vi "PH_SHS_Analysis.PC Set SHS Device Config.vi"(0 "i ref in":refnum<vi>, 2 "SHS Device Config":T1 {"wavelength [m]" format="%#_6p"; "pixel size [m/px]" format="%#_6p"; "focal length [m]" format="%#_6p"}, 5 "error IO":errorcluster) -> (14 "i ref out":refnum<vi>, 19 "error out":errorcluster)   [LabVIEW 2014, in "PH_SHS_Analysis.lvlib"]
uses:
  PH_SHS_Analysis.lvlib
  CSlibraries-extern/shs/SHS_Analysis/SHS_DeviceConfig.ctl
  CSlibraries-extern/shs/SHS_Analysis/SHS_Analysis.lvlib
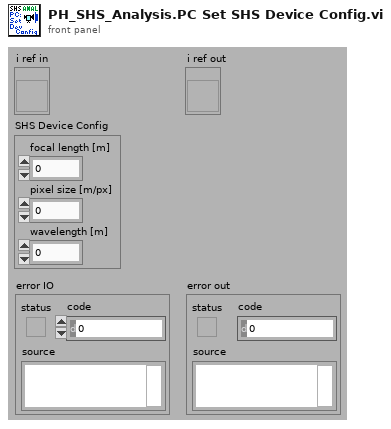
[diagram p1: front panel]
types:
  T1 = typedef "SHS_Analysis.lvlib/SHS_DeviceConfig.ctl" = cluster{"focal length [m]":dbl, "pixel size [m/px]":dbl, "wavelength [m]":dbl}
  T2 = typedef "PH_SHS_Analysis.lvlib/PH_SHS_Analysis.i attribute.ctl" = cluster{"GUI Refs":cluster{"Delete":refnum<vi>, "Global On":refnum<vi>, "Cam Source":refnum<vi>, "Calibration Data File":refnum<vi>, "Calibration status":refnum<vi>, "Show overlay":refnum<vi>, "SHS Device Config":refnum<vi>, "Result":refnum<vi>, "Consider Tilt":refnum<vi>, "Working Reference":refnum<vi>, "Remove Tilt":refnum<vi>, "Take Cali  Reference":refnum<vi>, "Publishing Data Status":refnum<vi>, "Calibration Data":refnum<vi>}, "Calibration":cluster{"Status":T3, "Data":T4, "File":path}, "Result":T9, "Image":T12, "SHS Device Config":T1, "Show Overlay":bool, "GradientZernikeMatrix":dbl[][], "Consider Tilt":bool, "Working Reference":T5, "Zernicke Service ID":i32, "PSDB Image":T12}
  T3 = typedef "PH_StatusHandler.lvlib/PH_StatusHandler.Status.ctl" = i16
  T4 = typedef "PH_SHS_Analysis_Calibrator.lvlib/PH_SHS_Analysis_Calibrator.Analysis Calibration Data.ctl" = cluster{"Date":string, "Time":string, "Cam Settings":cluster{"Cam ID":string, "Gain":dbl, "Brightness":dbl, "Shutter":dbl, "Cam Error":bool, "Mode":i32}, "SHS Reference Result":T5, "Pixel Size":dbl, "MLA Pitch":dbl, "Method":enum16{"automatic", "manual"}, "Calibration Data calculated":bool, "No Problems at calculation?":bool, "error out":errorcluster}
  T5 = typedef "SHS_Common.lvlib/SHSReference.ctl" = cluster{"Reference":T6[][], "Lens Array Pitch [px]":dbl}
  T6 = typedef "SHS_Common.lvlib/ReferencePoint.ctl" = cluster{"Rect":T7, "Point":T8}
  T7 = typedef "SHS_Common.lvlib/Rectangle.ctl" = cluster{"Left":i32, "Top":i32, "Right":i32, "Bottom":i32}
  T8 = typedef "SHS_Common.lvlib/Point.ctl" = cluster{"x":dbl, "y":dbl, "valid?":bool, "weight":dbl}
  T9 = typedef "PH_SHS_Analysis.lvlib/PH_SHS_Analysis.Result.ctl" = cluster{"Time Stamp":timestamp, "Zernike Coefficients":T10, "PtV [lambda]":dbl, "Shifts":T11, "Measurement Quality":cluster{dbl, dbl, dbl}, "Measurement valid?":bool}
  T10 = typedef "PH_SHS_Analysis.lvlib/PH_SHS_Analysis.Zernike Coefficients.ctl" = cluster{"Tilt x":dbl, "Tilt y":dbl, "Defocus":dbl, "Astig 0°":dbl, "Astig 45°":dbl, "Coma x":dbl, "Coma y":dbl, "Spherical":dbl, "Trefoil 0°":dbl, "Trefoil 30°":dbl, "2nd Astig 0°":dbl, "2nd Astig 45°":dbl, "2nd Coma x":dbl, "2nd Coma y":dbl, "2nd Spherical":dbl}
  T11 = typedef "SHS_Common.lvlib/Shifts.ctl" = T8[][]
  T12 = typedef "IMAQ Image.ctl" = refnum<image>
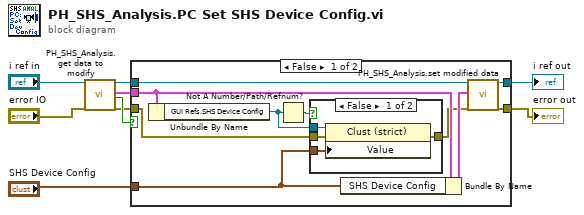
[diagram p0: block diagram]
diagram:
  n1 = call "PH_SHS_Analysis.get data to modify.vi"("i ref in"="i ref in", "error in (no error)"="error IO") -> ("i ref out"=w3:refnum<vi>, "i attribute"=w9:T2, "timed out"=w8:bool, "error out"=w2:errorcluster)  [unwired: 14 in]
  n2 = case shown="False" w8 {
    tunnel: w2 -> [w13 w25]
    tunnel: w3 -> [w19 w26]
    tunnel: [w18 w26] -> w5
    tunnel: [w17 w25] -> w7
    tunnel: w9 -> [w15 _]
    tunnel: "SHS Device Config" -> [w10 _]
    frame False {
      n3 = Unbundle By Name(w15) -> ("GUI Refs.SHS Device Config"=w11:refnum<vi>)
      n4 = Not A Number/Path/Refnum?(number/path/refnum=w11) -> (NaN/Path/Refnum?=w12:bool)
      n5 = case shown="False" w12 {
        tunnel: [w23 w24] -> w14
        tunnel: w11 -> [w22 _]
        tunnel: w10 -> [w21 _]
        tunnel: w13 -> [w20 w24]
        frame False {
          n6 = property class="Clust (strict)"(reference=w22, error in=w20, "Value"=w21) -> (error out=w23:errorcluster)  [unwired: 1 out]
        }
        frame True {
        }
      }
      n7 = Bundle By Name(cluster=w15, "SHS Device Config"=w10) -> (w16:T2)
      n8 = call "PH_SHS_Analysis.set modified data.vi"("i ref in"=w19, "i attribute"=w16, "error in (no error)"=w14) -> ("i ref out"=w18:refnum<vi>, "error out"=w17:errorcluster)  [unwired: 15 in]
    }
    frame True {
    }
  }
  "error out" <- w7
  "i ref out" <- w5
